vi "VISJS Viewer.vi"(4 "Extra Scripts":string, 5 "FileDependency In":map{path, T1}(c390), 6 "Options":string, 7 "OpenWebBrowser(False)":bool, 8 "error in":errorcluster, 9 "Embedd VISJS Librarya in HTMl File(False)":bool, 10 "HTMLFilePath":path, 11 "LibraryDependency":map{path, T3}(c390)) -> (0 "error out":errorcluster, 3 "HTMLFileContent":string)   [LabVIEW 2020, in "VISJS Viewer.lvlib"] (continued)
g.length>C&&e<=10;){e+=1;var o=g.length;if(e%3==0?this.body.modules.clustering.clusterBridges(I):this.body.modules.clustering.clusterOutliers(I),o==g.length&&e%3!=0)return this._declusterAll(),this.body.emitter.emit(\"_layoutFailed\"),void console.info(\"This network could not be positioned by this version of the improved layout algorithm. Please disable improvedLayout for better performance.\")}this.body.modules.kamadaKawai.setOptions({springLength:Math.max(150,2*i)})}e>10&&console.info(\"The clustering didn't succeed within the amount of interations allowed, progressing with partial result.\"),this.body.modules.kamadaKawai.solve(g,this.body.edgeIndices,!0),this._shiftToCenter();for(var n=0;n<g.length;n++){var r=this.body.nodes[g[n]];!1===r.predefinedPosition&&(r.x+=70*(.5-this._rng()),r.y+=70*(.5-this._rng()))}this._declusterAll(),this.body.emitter.emit(\"_repositionBezierNodes\")}}}},{key:\"_shiftToCenter\",value:function(){for(var g=XR.getRangeCore(this.body.nodes,this.body.nodeIndices),t=XR.findCenter(g),A=0;A<this.body.nodeIndices.length;A++){var e=this.body.nodes[this.body.nodeIndices[A]];e.x-=t.x,e.y-=t.y}}},{key:\"_declusterAll\",value:function(){for(var g=!0;!0===g;){g=!1;for(var t=0;t<this.body.nodeIndices.length;t++)!0===this.body.nodes[this.body.nodeIndices[t]].isCluster&&(g=!0,this.body.modules.clustering.openCluster(this.body.nodeIndices[t],{},!1));!0===g&&this.body.emitter.emit(\"_dataChanged\")}}},{key:\"getSeed\",value:function(){return this.initialRandomSeed}},{key:\"setupHierarchicalLayout\",value:function(){if(!0===this.options.hierarchical.enabled&&this.body.nodeIndices.length>0){var g,t,A=!1,e=!1;for(t in this.lastNodeOnLevel={},this.hierarchical=new SM,this.body.nodes)Object.prototype.hasOwnProperty.call(this.body.nodes,t)&&(void 0!==(g=this.body.nodes[t]).options.level?(A=!0,this.hierarchical.levels[t]=g.options.level):e=!0);if(!0===e&&!0===A)throw new Error(\"To use the hierarchical layout, nodes require either no predefined levels or levels have to be defined for all nodes.\");if(!0===e){var C=this.options.hierarchical.sortMethod;\"hubsize\"===C?this._determineLevelsByHubsize():\"directed\"===C?this._determineLevelsDirected():\"custom\"===C&&this._determineLevelsCustomCallback()}for(var I in this.body.nodes)Object.prototype.hasOwnProperty.call(this.body.nodes,I)&&this.hierarchical.ensureLevel(I);var i=this._getDistribution();this._generateMap(),this._placeNodesByHierarchy(i),this._condenseHierarchy(),this._shiftToCenter()}}},{key:\"_condenseHierarchy\",value:function(){var g=this,t=!1,A={},e=function(t,A){var e=g.hierarchical.trees;for(var C in e)Object.prototype.hasOwnProperty.call(e,C)&&e[C]===t&&g.direction.shift(C,A)},C=function(){for(var t=[],A=0;A<g.hierarchical.numTrees();A++)t.push(g.direction.getTreeSize(A));return t},I=function t(A,e){if(!e[A.id]&&(e[A.id]=!0,g.hierarchical.childrenReference[A.id])){var C=g.hierarchical.childrenReference[A.id];if(C.length>0)for(var I=0;I<C.length;I++)t(g.body.nodes[C[I]],e)}},i=function(t){var A=arguments.length>1&&void 0!==arguments[1]?arguments[1]:1e9,e=1e9,C=1e9,I=1e9,i=-1e9;for(var o in t)if(Object.prototype.hasOwnProperty.call(t,o)){var n=g.body.nodes[o],r=g.hierarchical.levels[n.id],s=g.direction.getPosition(n),a=lh(g._getSpaceAroundNode(n,t),2),d=a[0],h=a[1];e=Math.min(d,e),C=Math.min(h,C),r<=A&&(I=Math.min(s,I),i=Math.max(s,i))}return[I,i,e,C]},o=function(t,A,e){for(var C=g.hierarchical,I=0;I<A.length;I++){var i=A[I],o=C.distributionOrdering[i];if(o.length>1)for(var n=0;n<o.length-1;n++){var r=o[n],s=o[n+1];C.hasSameParent(r,s)&&C.inSameSubNetwork(r,s)&&t(r,s,e)}}},n=function(A,e){var C=arguments.length>2&&void 0!==arguments[2]&&arguments[2],o=g.direction.getPosition(A),n=g.direction.getPosition(e),r=Math.abs(n-o),s=g.options.hierarchical.nodeSpacing;if(r>s){var a={},d={};I(A,a),I(e,d);var h=function(t,A){var e=g.hierarchical.getMaxLevel(t.id),C=g.hierarchical.getMaxLevel(A.id);return Math.min(e,C)}(A,e),l=i(a,h),c=i(d,h),u=l[1],p=c[0],f=c[2];if(Math.abs(u-p)>s){var v=u-p+s;v<-f+s&&(v=-f+s),v<0&&(g._shiftBlock(e.id,v),t=!0,!0===C&&g._centerParent(e))}}},r=function(e,C){for(var o=C.id,n=C.edges,r=g.hierarchical.levels[C.id],s=g.options.hierarchical.levelSeparation*g.options.hierarchical.levelSeparation,a={},d=[],h=0;h<n.length;h++){var l=n[h];if(l.toId!=l.fromId){var c=l.toId==o?l.from:l.to;a[n[h].id]=c,g.hierarchical.levels[c.id]<r&&d.push(l)}}var u=function(t,A){for(var e=0,C=0;C<A.length;C++)if(void 0!==a[A[C].id]){var I=g.direction.getPosition(a[A[C].id])-t;e+=I/Math.sqrt(I*I+s)}return e},p=function(t,A){for(var e=0,C=0;C<A.length;C++)if(void 0!==a[A[C].id]){var I=g.direction.getPosition(a[A[C].id])-t;e-=s*Math.pow(I*I+s,-1.5)}return e},f=function(t,A){for(var e=g.direction.getPosition(C),I={},i=0;i<t;i++){var o=u(e,A),n=p(e,A);if(void 0!==I[e-=Math.max(-40,Math.min(40,Math.round(o/n)))])break;I[e]=i}return e},v=f(e,d);!function(e){var o=g.direction.getPosition(C);if(void 0===A[C.id]){var n={};I(C,n),A[C.id]=n}var r=i(A[C.id]),s=r[2],a=r[3],d=e-o,h=0;d>0?h=Math.min(d,a-g.options.hierarchical.nodeSpacing):d<0&&(h=-Math.min(-d,s-g.options.hierarchical.nodeSpacing)),0!=h&&(g._shiftBlock(C.id,h),t=!0)}(v),function(A){var e=g.direction.getPosition(C),I=lh(g._getSpaceAroundNode(C),2),i=I[0],o=I[1],n=A-e,r=e;n>0?r=Math.min(e+(o-g.options.hierarchical.nodeSpacing),A):n<0&&(r=Math.max(e-(i-g.options.hierarchical.nodeSpacing),A)),r!==e&&(g.direction.setPosition(C,r),t=!0)}(v=f(e,n))};!0===this.options.hierarchical.blockShifting&&(function(A){var e=g.hierarchical.getLevels();e=cl(e).call(e);for(var C=0;C<A&&(t=!1,o(n,e,!0),!0===t);C++);}(5),function(){for(var t in g.body.nodes)Object.prototype.hasOwnProperty.call(g.body.nodes,t)&&g._centerParent(g.body.nodes[t])}()),!0===this.options.hierarchical.edgeMinimization&&function(A){var e=g.hierarchical.getLevels();e=cl(e).call(e);for(var C=0;C<A;C++){t=!1;for(var I=0;I<e.length;I++)for(var i=e[I],o=g.hierarchical.distributionOrdering[i],n=0;n<o.length;n++)r(1e3,o[n]);if(!0!==t)break}}(20),!0===this.options.hierarchical.parentCentralization&&function(){var t=g.hierarchical.getLevels();t=cl(t).call(t);for(var A=0;A<t.length;A++)for(var e=t[A],C=g.hierarchical.distributionOrdering[e],I=0;I<C.length;I++)g._centerParent(C[I])}(),function(){for(var t=C(),A=0,I=0;I<t.length-1;I++){A+=t[I].max-t[I+1].min+g.options.hierarchical.treeSpacing,e(I+1,A)}}()}},{key:\"_getSpaceAroundNode\",value:function(g,t){var A=!0;void 0===t&&(A=!1);var e=this.hierarchical.levels[g.id];if(void 0!==e){var C=this.hierarchical.distributionIndex[g.id],I=this.direction.getPosition(g),i=this.hierarchical.distributionOrdering[e],o=1e9,n=1e9;if(0!==C){var r=i[C-1];if(!0===A&&void 0===t[r.id]||!1===A)o=I-this.direction.getPosition(r)}if(C!=i.length-1){var s=i[C+1];if(!0===A&&void 0===t[s.id]||!1===A){var a=this.direction.getPosition(s);n=Math.min(n,a-I)}}return[o,n]}return[0,0]}},{key:\"_centerParent\",value:function(g){if(this.hierarchical.parentReference[g.id])for(var t=this.hierarchical.parentReference[g.id],A=0;A<t.length;A++){var e=t[A],C=this.body.nodes[e],I=this.hierarchical.childrenReference[e];if(void 0!==I){var i=this._getCenterPosition(I),o=this.direction.getPosition(C),n=lh(this._getSpaceAroundNode(C),2),r=n[0],s=n[1],a=o-i;(a<0&&Math.abs(a)<s-this.options.hierarchical.nodeSpacing||a>0&&Math.abs(a)<r-this.options.hierarchical.nodeSpacing)&&this.direction.setPosition(C,i)}}}},{key:\"_placeNodesByHierarchy\",value:function(g){for(var t in this.positionedNodes={},g)if(Object.prototype.hasOwnProperty.call(g,t)){var A,e=Lh(g[t]);e=this._indexArrayToNodes(e),WO(A=this.direction).call(A,e);for(var C=0,I=0;I<e.length;I++){var i=e[I];if(void 0===this.positionedNodes[i.id]){var o=this.options.hierarchical.nodeSpacing,n=o*C;C>0&&(n=this.direction.getPosition(e[I-1])+o),this.direction.setPosition(i,n,t),this._validatePositionAndContinue(i,t,n),C++}}}}},{key:\"_placeBranchNodes\",value:function(g,t){var A,e=this.hierarchical.childrenReference[g];if(void 0!==e){for(var C=[],I=0;I<e.length;I++)C.push(this.body.nodes[e[I]]);WO(A=this.direction).call(A,C);for(var i=0;i<C.length;i++){var o=C[i],n=this.hierarchical.levels[o.id];if(!(n>t&&void 0===this.positionedNodes[o.id]))return;var r=this.options.hierarchical.nodeSpacing,s=void 0;s=0===i?this.direction.getPosition(this.body.nodes[g]):this.direction.getPosition(C[i-1])+r,this.direction.setPosition(o,s,n),this._validatePositionAndContinue(o,n,s)}var a=this._getCenterPosition(C);this.direction.setPosition(this.body.nodes[g],a,t)}}},{key:\"_validatePositionAndContinue\",value:function(g,t,A){if(this.hierarchical.isTree){if(void 0!==this.lastNodeOnLevel[t]){var e=this.direction.getPosition(this.body.nodes[this.lastNodeOnLevel[t]]);if(A-e<this.options.hierarchical.nodeSpacing){var C=e+this.options.hierarchical.nodeSpacing-A,I=this._findCommonParent(this.lastNodeOnLevel[t],g.id);this._shiftBlock(I.withChild,C)}}this.lastNodeOnLevel[t]=g.id,this.positionedNodes[g.id]=!0,this._placeBranchNodes(g.id,t)}}},{key:\"_indexArrayToNodes\",value:function(g){for(var t=[],A=0;A<g.length;A++)t.push(this.body.nodes[g[A]]);return t}},{key:\"_getDistribution\",value:function(){var g,t,A={};for(g in this.body.nodes)if(Object.prototype.hasOwnProperty.call(this.body.nodes,g)){t=this.body.nodes[g];var e=void 0===this.hierarchical.levels[g]?0:this.hierarchical.levels[g];this.direction.fix(t,e),void 0===A[e]&&(A[e]={}),A[e][g]=t}return A}},{key:\"_getActiveEdges\",value:function(g){var t=this,A=[];return tv(g.edges,(function(g){var e;-1!==Xc(e=t.body.edgeIndices).call(e,g.id)&&A.push(g)})),A}},{key:\"_getHubSizes\",value:function(){var g=this,t={};tv(this.body.nodeIndices,(function(A){var e=g.body.nodes[A],C=g._getActiveEdges(e).length;t[C]=!0}));var A=[];return tv(t,(function(g){A.push(Number(g))})),WO(A).call(A,(function(g,t){return t-g})),A}},{key:\"_determineLevelsByHubsize\",value:function(){for(var g=this,t=function(t,A){g.hierarchical.levelDownstream(t,A)},A=this._getHubSizes(),e=function(){var e=A[C];if(0===e)return 1;tv(g.body.nodeIndices,(function(A){var C=g.body.nodes[A];e===g._getActiveEdges(C).length&&g._crawlNetwork(t,A)}))},C=0;C<A.length&&!e();++C);}},{key:\"_determineLevelsCustomCallback\",value:function(){var g=this;this._crawlNetwork((function(t,A,e){var C=g.hierarchical.levels[t.id];void 0===C&&(C=g.hierarchical.levels[t.id]=1e5);var I=(XR.cloneOptions(t,\"node\"),XR.cloneOptions(A,\"node\"),void XR.cloneOptions(e,\"edge\"));g.hierarchical.levels[A.id]=C+I})),this.hierarchical.setMinLevelToZero(this.body.nodes)}},{key:\"_determineLevelsDirected\",value:function(){var g,t=this,A=LE(g=this.body.nodeIndices).call(g,(function(g,A){return g.set(A,t.body.nodes[A]),g}),new Fm);\"roots\"===this.options.hierarchical.shakeTowards?this.hierarchical.levels=function(g){return zM((function(t){var A,e;return RM(A=pc(e=t.edges).call(e,(function(t){return g.has(t.toId)}))).call(A,(function(g){return g.from===t}))}),(function(g,t){return t<g}),\"to\",g)}(A):this.hierarchical.levels=function(g){return zM((function(t){var A,e;return RM(A=pc(e=t.edges).call(e,(function(t){return g.has(t.toId)}))).call(A,(function(g){return g.to===t}))}),(function(g,t){return t>g}),\"from\",g)}(A),this.hierarchical.setMinLevelToZero(this.body.nodes)}},{key:\"_generateMap\",value:function(){var g=this;this._crawlNetwork((function(t,A){g.hierarchical.levels[A.id]>g.hierarchical.levels[t.id]&&g.hierarchical.addRelation(t.id,A.id)})),this.hierarchical.checkIfTree()}},{key:\"_crawlNetwork\",value:function(){var g=this,t=arguments.length>0&&void 0!==arguments[0]?arguments[0]:function(){},A=arguments.length>1?arguments[1]:void 0,e={},C=function A(C,I){if(void 0===e[C.id]){var i;g.hierarchical.setTreeIndex(C,I),e[C.id]=!0;for(var o=g._getActiveEdges(C),n=0;n<o.length;n++){var r=o[n];!0===r.connected&&(i=r.toId==C.id?r.from:r.to,C.id!=i.id&&(t(C,i,r),A(i,I)))}}};if(void 0===A)for(var I=0,i=0;i<this.body.nodeIndices.length;i++){var o=this.body.nodeIndices[i];if(void 0===e[o])C(this.body.nodes[o],I),I+=1}else{var n=this.body.nodes[A];if(void 0===n)return void console.error(\"Node not found:\",A);C(n)}}},{key:\"_shiftBlock\",value:function(g,t){var A=this,e={};!function g(C){if(!e[C]){e[C]=!0,A.direction.shift(C,t);var I=A.hierarchical.childrenReference[C];if(void 0!==I)for(var i=0;i<I.length;i++)g(I[i])}}(g)}},{key:\"_findCommonParent\",value:function(g,t){var A=this,e={};return function g(t,e){var C=A.hierarchical.parentReference[e];if(void 0!==C)for(var I=0;I<C.length;I++){var i=C[I];t[i]=!0,g(t,i)}}(e,g),function g(t,e){var C=A.hierarchical.parentReference[e];if(void 0!==C)for(var I=0;I<C.length;I++){var i=C[I];if(void 0!==t[i])return{foundParent:i,withChild:e};var o=g(t,i);if(null!==o.foundParent)return o}return{foundParent:null,withChild:e}}(e,t)}},{key:\"setDirectionStrategy\",value:function(){var g=\"UD\"===this.options.hierarchical.direction||\"DU\"===this.options.hierarchical.direction;this.direction=g?new wM(this):new kM(this)}},{key:\"_getCenterPosition\",value:function(g){for(var t=1e9,A=-1e9,e=0;e<g.length;e++){var C=void 0;if(void 0!==g[e].id)C=g[e];else{var I=g[e];C=this.body.nodes[I]}var i=this.direction.getPosition(C);t=Math.min(t,i),A=Math.max(A,i)}return.5*(t+A)}}]),g}();function FM(g,t){var A=void 0!==uh&&ln(g)||g[\"@@iterator\"];if(!A){if(Rh(g)||(A=function(g,t){var A;if(!g)return;if(\"string\"==typeof g)return GM(g,t);var e=wh(A=Object.prototype.toString.call(g)).call(A,8,-1);\"Object\"===e&&g.constructor&&(e=g.constructor.name);if(\"Map\"===e||\"Set\"===e)return Uo(g);if(\"Arguments\"===e||/^(?:Ui|I)nt(?:8|16|32)(?:Clamped)?Array$/.test(e))return GM(g,t)}(g))||t&&g&&\"number\"==typeof g.length){A&&(g=A);var e=0,C=function(){};return{s:C,n:function(){return e>=g.length?{done:!0}:{done:!1,value:g[e++]}},e:function(g){throw g},f:C}}throw new TypeError(\"Invalid attempt to iterate non-iterable instance.\\nIn order to be iterable, non-array objects must have a [Symbol.iterator]() method.\")}var I,i=!0,o=!1;return{s:function(){A=A.call(g)},n:function(){var g=A.next();return i=g.done,g},e:function(g){o=!0,I=g},f:function(){try{i||null==A.return||A.return()}finally{if(o)throw I}}}}function GM(g,t){(null==t||t>g.length)&&(t=g.length);for(var A=0,e=new Array(t);A<t;A++)e[A]=g[A];return e}_e('div.vis-network div.vis-manipulation{background:#fff;background:-moz-linear-gradient(top,#fff 0,#fcfcfc 48%,#fafafa 50%,#fcfcfc 100%);background:-webkit-gradient(linear,left top,left bottom,color-stop(0,#fff),color-stop(48%,#fcfcfc),color-stop(50%,#fafafa),color-stop(100%,#fcfcfc));background:-webkit-linear-gradient(top,#fff,#fcfcfc 48%,#fafafa 50%,#fcfcfc);background:-o-linear-gradient(top,#fff 0,#fcfcfc 48%,#fafafa 50%,#fcfcfc 100%);background:-ms-linear-gradient(top,#fff 0,#fcfcfc 48%,#fafafa 50%,#fcfcfc 100%);background:linear-gradient(180deg,#fff 0,#fcfcfc 48%,#fafafa 50%,#fcfcfc);border:0 solid #d6d9d8;border-bottom:1px;box-sizing:content-box;filter:progid:DXImageTransform.Microsoft.gradient(startColorstr=\"#ffffff\",endColorstr=\"#fcfcfc\",GradientType=0);height:28px;left:0;padding-top:4px;position:absolute;top:0;width:100%}div.vis-network button.vis-edit-mode,div.vis-network div.vis-edit-mode{height:30px;left:0;position:absolute;top:5px}div.vis-network button.vis-close{-webkit-touch-callout:none;background-color:transparent;background-image:url(\"data:image/png;base64,iVBORw0KGgoAAAANSUhEUgAAAAcAAAAHCAYAAADEUlfTAAAACXBIWXMAAAsTAAALEwEAmpwYAAAKT2lDQ1BQaG90b3Nob3AgSUNDIHByb2ZpbGUAAHjanVNnVFPpFj333vRCS4iAlEtvUhUIIFJCi4AUkSYqIQkQSoghodkVUcERRUUEG8igiAOOjoCMFVEsDIoK2AfkIaKOg6OIisr74Xuja9a89+bN/rXXPues852zzwfACAyWSDNRNYAMqUIeEeCDx8TG4eQuQIEKJHAAEAizZCFz/SMBAPh+PDwrIsAHvgABeNMLCADATZvAMByH/w/qQplcAYCEAcB0kThLCIAUAEB6jkKmAEBGAYCdmCZTAKAEAGDLY2LjAFAtAGAnf+bTAICd+Jl7AQBblCEVAaCRACATZYhEAGg7AKzPVopFAFgwABRmS8Q5ANgtADBJV2ZIALC3AMDOEAuyAAgMADBRiIUpAAR7AGDIIyN4AISZABRG8lc88SuuEOcqAAB4mbI8uSQ5RYFbCC1xB1dXLh4ozkkXKxQ2YQJhmkAuwnmZGTKBNA/g88wAAKCRFRHgg/P9eM4Ors7ONo62Dl8t6r8G/yJiYuP+5c+rcEAAAOF0ftH+LC+zGoA7BoBt/qIl7gRoXgugdfeLZrIPQLUAoOnaV/Nw+H48PEWhkLnZ2eXk5NhKxEJbYcpXff5nwl/AV/1s+X48/Pf14L7iJIEyXYFHBPjgwsz0TKUcz5IJhGLc5o9H/LcL//wd0yLESWK5WCoU41EScY5EmozzMqUiiUKSKcUl0v9k4t8s+wM+3zUAsGo+AXuRLahdYwP2SycQWHTA4vcAAPK7b8HUKAgDgGiD4c93/+8//UegJQCAZkmScQAAXkQkLlTKsz/HCAAARKCBKrBBG/TBGCzABhzBBdzBC/xgNoRCJMTCQhBCCmSAHHJgKayCQiiGzbAdKmAv1EAdNMBRaIaTcA4uwlW4Dj1wD/phCJ7BKLyBCQRByAgTYSHaiAFiilgjjggXmYX4IcFIBBKLJCDJiBRRIkuRNUgxUopUIFVIHfI9cgI5h1xGupE7yAAygvyGvEcxlIGyUT3UDLVDuag3GoRGogvQZHQxmo8WoJvQcrQaPYw2oefQq2gP2o8+Q8cwwOgYBzPEbDAuxsNCsTgsCZNjy7EirAyrxhqwVqwDu4n1Y8+xdwQSgUXACTYEd0IgYR5BSFhMWE7YSKggHCQ0EdoJNwkDhFHCJyKTqEu0JroR+cQYYjIxh1hILCPWEo8TLxB7iEPENyQSiUMyJ7mQAkmxpFTSEtJG0m5SI+ksqZs0SBojk8naZGuyBzmULCAryIXkneTD5DPkG+Qh8lsKnWJAcaT4U+IoUspqShnlEOU05QZlmDJBVaOaUt2ooVQRNY9aQq2htlKvUYeoEzR1mjnNgxZJS6WtopXTGmgXaPdpr+h0uhHdlR5Ol9BX0svpR+iX6AP0dwwNhhWDx4hnKBmbGAcYZxl3GK+YTKYZ04sZx1QwNzHrmOeZD5lvVVgqtip8FZHKCpVKlSaVGyovVKmqpqreqgtV81XLVI+pXlN9rkZVM1PjqQnUlqtVqp1Q61MbU2epO6iHqmeob1Q/pH5Z/YkGWcNMw09DpFGgsV/jvMYgC2MZs3gsIWsNq4Z1gTXEJrHN2Xx2KruY/R27iz2qqaE5QzNKM1ezUvOUZj8H45hx+Jx0TgnnKKeX836K3hTvKeIpG6Y0TLkxZVxrqpaXllirSKtRq0frvTau7aedpr1Fu1n7gQ5Bx0onXCdHZ4/OBZ3nU9lT3acKpxZNPTr1ri6qa6UbobtEd79up+6Ynr5egJ5Mb6feeb3n+hx9L/1U/W36p/VHDFgGswwkBtsMzhg8xTVxbzwdL8fb8VFDXcNAQ6VhlWGX4YSRudE8o9VGjUYPjGnGXOMk423GbcajJgYmISZLTepN7ppSTbmmKaY7TDtMx83MzaLN1pk1mz0x1zLnm+eb15vft2BaeFostqi2uGVJsuRaplnutrxuhVo5WaVYVVpds0atna0l1rutu6cRp7lOk06rntZnw7Dxtsm2qbcZsOXYBtuutm22fWFnYhdnt8Wuw+6TvZN9un2N/T0HDYfZDqsdWh1+c7RyFDpWOt6azpzuP33F9JbpL2dYzxDP2DPjthPLKcRpnVOb00dnF2e5c4PziIuJS4LLLpc+Lpsbxt3IveRKdPVxXeF60vWdm7Obwu2o26/uNu5p7ofcn8w0nymeWTNz0MPIQ+BR5dE/C5+VMGvfrH5PQ0+BZ7XnIy9jL5FXrdewt6V3qvdh7xc+9j5yn+M+4zw33jLeWV/MN8C3yLfLT8Nvnl+F30N/I/9k/3r/0QCngCUBZwOJgUGBWwL7+Hp8Ib+OPzrbZfay2e1BjKC5QRVBj4KtguXBrSFoyOyQrSH355jOkc5pDoVQfujW0Adh5mGLw34MJ4WHhVeGP45wiFga0TGXNXfR3ENz30T6RJZE3ptnMU85ry1KNSo+qi5qPNo3ujS6P8YuZlnM1VidWElsSxw5LiquNm5svt/87fOH4p3iC+N7F5gvyF1weaHOwvSFpxapLhIsOpZATIhOOJTwQRAqqBaMJfITdyWOCnnCHcJnIi/RNtGI2ENcKh5O8kgqTXqS7JG8NXkkxTOlLOW5hCepkLxMDUzdmzqeFpp2IG0yPTq9MYOSkZBxQqohTZO2Z+pn5mZ2y6xlhbL+xW6Lty8elQfJa7OQrAVZLQq2QqboVFoo1yoHsmdlV2a/zYnKOZarnivN7cyzytuQN5zvn//tEsIS4ZK2pYZLVy0dWOa9rGo5sjxxedsK4xUFK4ZWBqw8uIq2Km3VT6vtV5eufr0mek1rgV7ByoLBtQFr6wtVCuWFfevc1+1dT1gvWd+1YfqGnRs+FYmKrhTbF5cVf9go3HjlG4dvyr+Z3JS0qavEuWTPZtJm6ebeLZ5bDpaql+aXDm4N2dq0Dd9WtO319kXbL5fNKNu7g7ZDuaO/PLi8ZafJzs07P1SkVPRU+lQ27tLdtWHX+G7R7ht7vPY07NXbW7z3/T7JvttVAVVN1WbVZftJ+7P3P66Jqun4lvttXa1ObXHtxwPSA/0HIw6217nU1R3SPVRSj9Yr60cOxx++/p3vdy0NNg1VjZzG4iNwRHnk6fcJ3/ceDTradox7rOEH0x92HWcdL2pCmvKaRptTmvtbYlu6T8w+0dbq3nr8R9sfD5w0PFl5SvNUyWna6YLTk2fyz4ydlZ19fi753GDborZ752PO32oPb++6EHTh0kX/i+c7vDvOXPK4dPKy2+UTV7hXmq86X23qdOo8/pPTT8e7nLuarrlca7nuer21e2b36RueN87d9L158Rb/1tWeOT3dvfN6b/fF9/XfFt1+cif9zsu72Xcn7q28T7xf9EDtQdlD3YfVP1v+3Njv3H9qwHeg89HcR/cGhYPP/pH1jw9DBY+Zj8uGDYbrnjg+OTniP3L96fynQ89kzyaeF/6i/suuFxYvfvjV69fO0ZjRoZfyl5O/bXyl/erA6xmv28bCxh6+yXgzMV70VvvtwXfcdx3vo98PT+R8IH8o/2j5sfVT0Kf7kxmTk/8EA5jz/GMzLdsAADvGaVRYdFhNTDpjb20uYWRvYmUueG1wAAAAAAA8P3hwYWNrZXQgYmVnaW49Iu+7vyIgaWQ9Ilc1TTBNcENlaGlIenJlU3pOVGN6a2M5ZCI/Pgo8eDp4bXBtZXRhIHhtbG5zOng9ImFkb2JlOm5zOm1ldGEvIiB4OnhtcHRrPSJBZG9iZSBYTVAgQ29yZSA1LjUtYzAyMSA3OS4xNTQ5MTEsIDIwMTMvMTAvMjktMTE6NDc6MTYgICAgICAgICI+CiAgIDxyZGY6UkRGIHhtbG5zOnJkZj0iaHR0cDovL3d3dy53My5vcmcvMTk5OS8wMi8yMi1yZGYtc3ludGF4LW5zIyI+CiAgICAgIDxyZGY6RGVzY3JpcHRpb24gcmRmOmFib3V0PSIiCiAgICAgICAgICAgIHhtbG5zOnhtcD0iaHR0cDovL25zLmFkb2JlLmNvbS94YXAvMS4wLyIKICAgICAgICAgICAgeG1sbnM6eG1wTU09Imh0dHA6Ly9ucy5hZG9iZS5jb20veGFwLzEuMC9tbS8iCiAgICAgICAgICAgIHhtbG5zOnN0RXZ0PSJodHRwOi8vbnMuYWRvYmUuY29tL3hhcC8xLjAvc1R5cGUvUmVzb3VyY2VFdmVudCMiCiAgICAgICAgICAgIHhtbG5zOmRjPSJodHRwOi8vcHVybC5vcmcvZGMvZWxlbWVudHMvMS4xLyIKICAgICAgICAgICAgeG1sbnM6cGhvdG9zaG9wPSJodHRwOi8vbnMuYWRvYmUuY29tL3Bob3Rvc2hvcC8xLjAvIgogICAgICAgICAgICB4bWxuczp0aWZmPSJodHRwOi8vbnMuYWRvYmUuY29tL3RpZmYvMS4wLyIKICAgICAgICAgICAgeG1sbnM6ZXhpZj0iaHR0cDovL25zLmFkb2JlLmNvbS9leGlmLzEuMC8iPgogICAgICAgICA8eG1wOkNyZWF0b3JUb29sPkFkb2JlIFBob3Rvc2hvcCBDQyAoV2luZG93cyk8L3htcDpDcmVhdG9yVG9vbD
